vi "SetQMC_SetQMCA.vi"(0 "System no.":i32=1 min=1 step=1, 1 "Function":enum16{"SetQMC", "SetQMCA"}(ring), 2 "Axis":u8, 3 "Command":u8, 5 "error in":errorcluster, 6 "Parameter":i32, 8 "Parameter 1":u16, 9 "Parameter 2":i32) -> (14 "DLL I32 Return value":i32, 19 "error out":errorcluster)   [LabVIEW 2026]
doc: "This VI calls the SetQMC or SetQMCA function in the GCSTranslator.dll. GCSTranslator.dll and the corresponding system specific GCS DLL must be installed. The VI reads the system name from Global 2 and calls the corresponding DLL function. Parameter is only valid for SetQMC, Parameter 1 and Parameter 2 are only valid for SetQMCA. When using as a sub-VI, take special care to use the correct data representation when connecting values to the input terminals. If coercion dots appear at the terminals, the VI may not function correctly. After changing values, the update function must be called to activate the new values. See user manual for details."
uses:
  Global1.vi
  GeneralCommands/Global2 (Array).vi
panel:
  # "This vi calls the SetQMC or SetQMCA function from \nGCSTranslator.dll. GCSTranslator.dll and the corresponding \nsystem specific GCS DLL must be installed. The VI reads \nthe system name from Global 2 and calls the corresponding \nDLL function. Parameter is only valid for SetQMC, Parameter\n1 and Parameter 2 are only valid for SetQMCA."
  # "General inputs:"
  # "Function specific inputs:"
  # "Only valid for SetQMC:"
  # "Only valid for SetQMCA:"
  # "Error handling:"
  # "DLL output:"
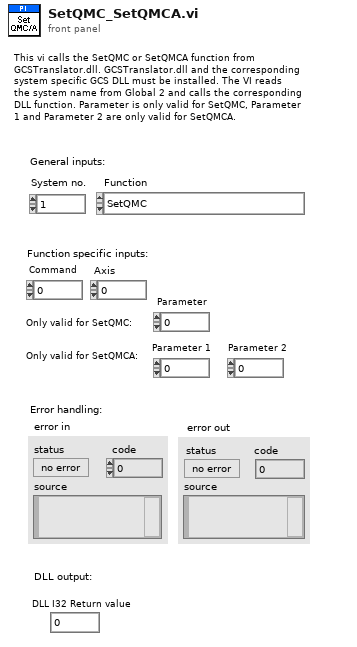
[diagram p1: front panel]
types:
  T1 = typedef "Controller names.ctl" = enum16{"None", "Analog", "C-702", "C-413", "C-414", "C-843", "C-843.PM", "C-844", "C-848", "C-865", "C-866", "C-867", "C-877", "C-880", "C-884", "C-885", "C-886", "C-887", "C-891", "E-135", "E-516", "E-517", "E-518", "E-709", "E-710", "E-712", "E-725", "E-727", "E-753", "E-754", "E-755", "E-761", "E-816", "E-861", "E-870", "E-871", "E-872", "E-873", "E-874", "F-206", "HydraPollux", "M-840", "M-850", "M-8X0", "Mercury", "Mercury_GCS", "PI_GCS2"}
  T2 = cluster{"Conn. axes":string[], "Controller name":T1}[]
  T3 = cluster{"Conn. axes":string[], "Controller name":T1}
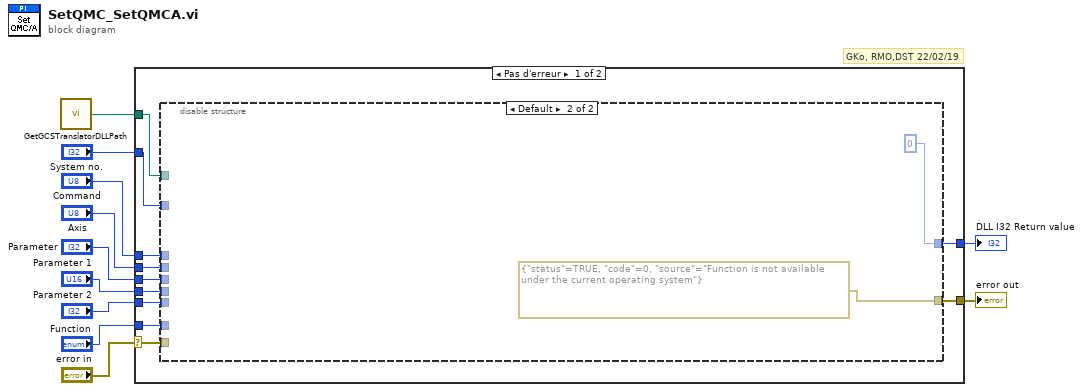
[diagram p0: block diagram]
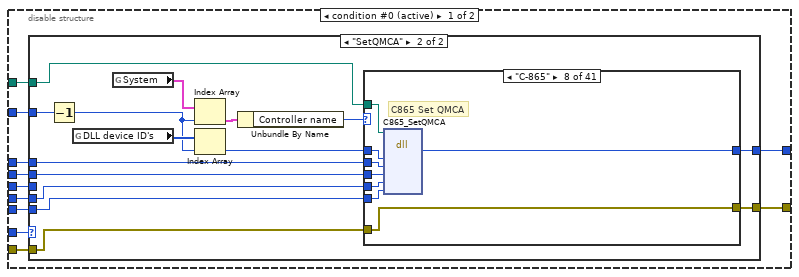
[diagram p2: hidden frame]
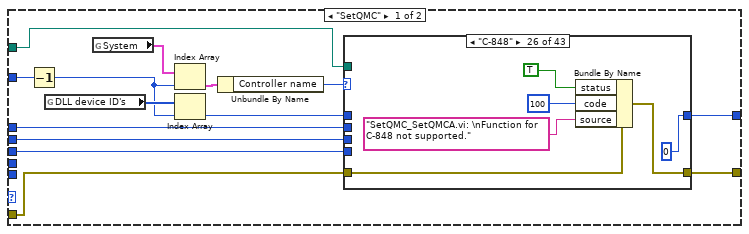
[diagram p3: hidden frame]
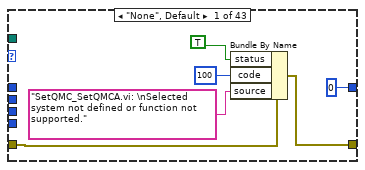
[diagram p4: hidden frame]
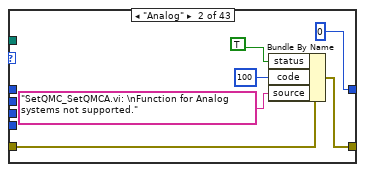
[diagram p5: hidden frame]
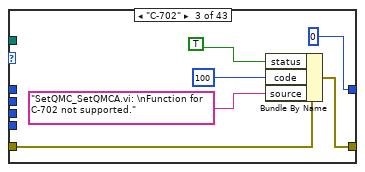
[diagram p6: hidden frame]
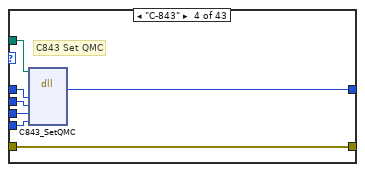
[diagram p7: hidden frame]
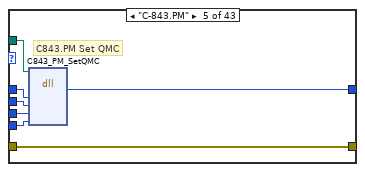
[diagram p8: hidden frame]
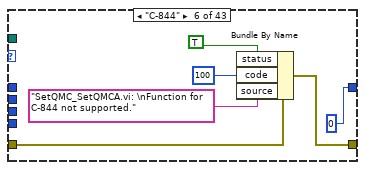
[diagram p9: hidden frame]
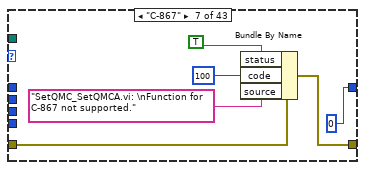
[diagram p10: hidden frame]
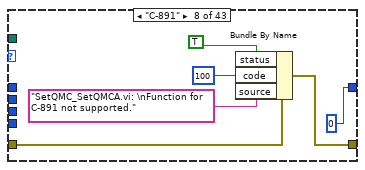
[diagram p11: hidden frame]
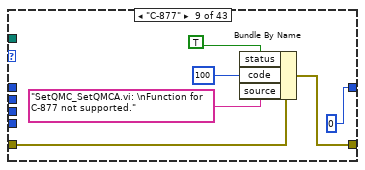
[diagram p12: hidden frame]
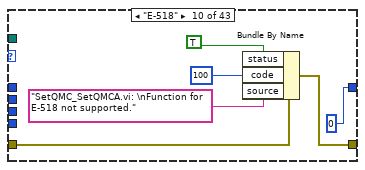
[diagram p13: hidden frame]
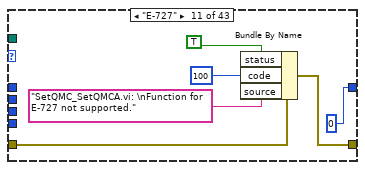
[diagram p14: hidden frame]
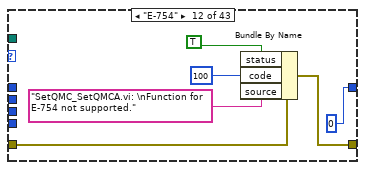
[diagram p15: hidden frame]
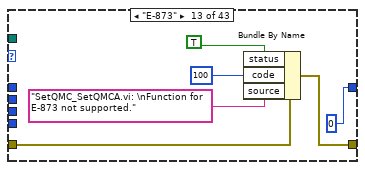
[diagram p16: hidden frame]
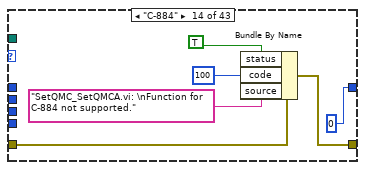
[diagram p17: hidden frame]
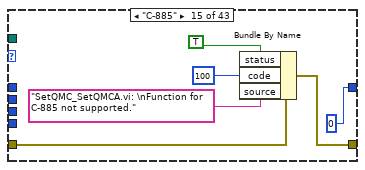
[diagram p18: hidden frame]
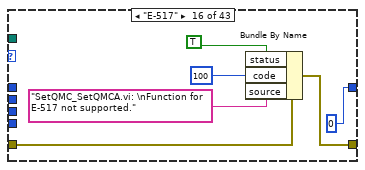
[diagram p19: hidden frame]
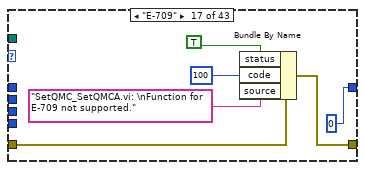
[diagram p20: hidden frame]
diagram:
  # "GKo, RMO,DST 22/02/19"
  n1 = call "GetGCSTranslatorDLLPath.vi"() -> ("DLL path"=w1:path)  [unwired: 1 in]
  n2 = case shown="Pas d'erreur" "error in" {
    selector: "error in" -> [w15 w581]
    tunnel: [w22 w581] -> w11
    tunnel: [w21 0] -> w10
    tunnel: "Command" -> [w20 _]
    tunnel: "Axis" -> [w19 _]
    tunnel: "Parameter" -> [w18 _]
    tunnel: "Parameter 1" -> [w17 _]
    tunnel: "Parameter 2" -> [w16 _]
    tunnel: "System no." -> [w14 _]
    tunnel: "Function" -> [w13 _]
    tunnel: w1 -> [w12 _]
    frame No Error {
      n3 = disable-structure shown="Default" {
        disable-tunnel: w13 -> [w33 _]
        disable-tunnel: [w32 errorcluster {"status"=TRUE, "code"=0, "source"="Function is not available under the current operating system"} ("error IO")] -> w22
        disable-tunnel: [w31 0] -> w21
        disable-tunnel: w14 -> [w30 _]
        disable-tunnel: w20 -> [w29 _]
        disable-tunnel: w19 -> [w28 _]
        disable-tunnel: w18 -> [w27 _]
        disable-tunnel: w17 -> [w26 _]
        disable-tunnel: w16 -> [w25 _]
        disable-tunnel: w15 -> [w24 _]
        disable-tunnel: w12 -> [w23 _]
        frame condition #0 (active) {
          n4 = case shown="\"SetQMCA\"" w33 {
            tunnel: w30 -> [w46 w323]
            tunnel: w24 -> [w40 w316]
            tunnel: [w39 w315] -> w32
            tunnel: [w47 w324] -> w31
            tunnel: w29 -> [w43 w320]
            tunnel: w28 -> [w42 w319]
            tunnel: w27 -> [w41 _]
            tunnel: w26 -> [_ w318]
            tunnel: w25 -> [_ w317]
            tunnel: w23 -> [w34 w310]
            frame "SetQMC" {
              n5 = Decrement(x=w46) -> (x-1=w37:i32)
              n6 = global read "Global1.vi" "DLL device ID's"() -> (w45:i32[])
              n7 = global read "Global2 (Array).vi" "System"() -> (w38:T2)
              n8 = Index Array(array=w38, index=w37) -> (element=w36:T3)
              n9 = Index Array(array=w45, index=w37) -> (element=w44:i32)
              n10 = Unbundle By Name(w36) -> ("Controller name"=w35:T1)
              n11 = case shown="\"C-848\"" w35 {
                tunnel: [0 0 0 w72 w79 0 0 0 0 0 0 0 0 0 0 0 0 0 0 0 0 0 0 0 0 0 w212 w219 0 0 0 0 0 0 0 0 0 0 0 0 0 0 0] -> w47
                tunnel: w44 -> [_ _ _ w71 w78 _ _ _ _ _ _ _ _ _ _ _ _ _ _ _ _ _ _ _ _ _ w211 w218 _ _ _ _ _ _ _ _ _ _ _ _ _ _ _]
                tunnel: w43 -> [_ _ _ w70 w77 _ _ _ _ _ _ _ _ _ _ _ _ _ _ _ _ _ _ _ _ _ w210 w217 _ _ _ _ _ _ _ _ _ _ _ _ _ _ _]
                tunnel: w42 -> [_ _ _ w69 w76 _ _ _ _ _ _ _ _ _ _ _ _ _ _ _ _ _ _ _ _ _ w209 w216 _ _ _ _ _ _ _ _ _ _ _ _ _ _ _]
                tunnel: w41 -> [_ _ _ w68 w75 _ _ _ _ _ _ _ _ _ _ _ _ _ _ _ _ _ _ _ _ _ w208 w215 _ _ _ _ _ _ _ _ _ _ _ _ _ _ _]
                tunnel: [w51 w58 w63 w67 w74 w83 w89 w95 w101 w107 w113 w119 w125 w131 w137 w143 w149 w155 w161 w167 w173 w179 w185 w191 w197 w203 w207 w214 w223 w229 w235 w241 w247 w253 w259 w265 w271 w277 w283 w289 w295 w301 w307] -> w39
                tunnel: w40 -> [w52 w54 w64 w67 w74 w84 w90 w96 w102 w108 w114 w120 w126 w132 w138 w144 w150 w156 w162 w168 w174 w180 w186 w192 w198 w204 w207 w214 w224 w230 w236 w242 w248 w254 w260 w266 w272 w278 w284 w290 w296 w302 w308]
                tunnel: w34 -> [_ _ _ w66 w73 _ _ _ _ _ _ _ _ _ _ _ _ _ _ _ _ _ _ _ _ _ w206 w213 _ _ _ _ _ _ _ _ _ _ _ _ _ _ _]
                frame "None", Default {
                  n12 = Bundle By Name(cluster=w52, "status"=TRUE, "code"=100, "source"="SetQMC_SetQMCA.vi: \nSelected system not defined or function not supported.") -> (w51:errorcluster)
                }
                frame "Analog" {
                  n13 = Bundle By Name(cluster=w54, "status"=TRUE, "code"=100, "source"="SetQMC_SetQMCA.vi: \nFunction for Analog systems not supported.") -> (w58:errorcluster)
                }
                frame "C-702" {
                  n14 = Bundle By Name(cluster=w64, "status"=TRUE, "code"=100, "source"="SetQMC_SetQMCA.vi: \nFunction for C-702 not supported.") -> (w63:errorcluster)
                }
                frame "C-843" {
                  # "C843 Set QMC"
                  n15 = dll-call lib="T:/Entwicklung/HostSoftware/LabVIEW/GCSDrivers/source/GCS2LabVIEW/Low Level/GCSTranslator.dll" fn="C843_SetQMC"(path in=w66, "ID"=w71, "Cmd"=w70, "Axis"=w69, "Param"=w68) -> ("return type"=w72:i32)  [unwired: 6 in, 2 out]
                }
                frame "C-843.PM" {
                  # "C843.PM Set QMC"
                  n16 = dll-call lib="T:/Entwicklung/HostSoftware/LabVIEW/GCSDrivers/source/GCS2LabVIEW/Low Level/GCSTranslator.dll" fn="C843_PM_SetQMC"(path in=w73, "ID"=w78, "Cmd"=w77, "Axis"=w76, "Param"=w75) -> ("return type"=w79:i32)  [unwired: 6 in, 2 out]
                }
                frame "C-844" {
                  n17 = Bundle By Name(cluster=w84, "status"=TRUE, "code"=100, "source"="SetQMC_SetQMCA.vi: \nFunction for C-844 not supported.") -> (w83:errorcluster)
                }
                frame "C-867" {
                  n18 = Bundle By Name(cluster=w90, "status"=TRUE, "code"=100, "source"="SetQMC_SetQMCA.vi: \nFunction for C-867 not supported.") -> (w89:errorcluster)
                }
                frame "C-891" {
                  n19 = Bundle By Name(cluster=w96, "status"=TRUE, "code"=100, "source"="SetQMC_SetQMCA.vi: \nFunction for C-891 not supported.") -> (w95:errorcluster)
                }
                frame "C-877" {
                  n20 = Bundle By Name(cluster=w102, "status"=TRUE, "code"=100, "source"="SetQMC_SetQMCA.vi: \nFunction for C-877 not supported.") -> (w101:errorcluster)
                }
                frame "E-518" {
                  n21 = Bundle By Name(cluster=w108, "status"=TRUE, "code"=100, "source"="SetQMC_SetQMCA.vi: \nFunction for E-518 not supported.") -> (w107:errorcluster)
                }
                frame "E-727" {
                  n22 = Bundle By Name(cluster=w114, "status"=TRUE, "code"=100, "source"="SetQMC_SetQMCA.vi: \nFunction for E-727 not supported.") -> (w113:errorcluster)
                }
                frame "E-754" {
                  n23 = Bundle By Name(cluster=w120, "status"=TRUE, "code"=100, "source"="SetQMC_SetQMCA.vi: \nFunction for E-754 not supported.") -> (w119:errorcluster)
                }
                frame "E-873" {
                  n24 = Bundle By Name(cluster=w126, "status"=TRUE, "code"=100, "source"="SetQMC_SetQMCA.vi: \nFunction for E-873 not supported.") -> (w125:errorcluster)
                }
                frame "C-884" {
                  n25 = Bundle By Name(cluster=w132, "status"=TRUE, "code"=100, "source"="SetQMC_SetQMCA.vi: \nFunction for C-884 not supported.") -> (w131:errorcluster)
                }
                frame "C-885" {
                  n26 = Bundle By Name(cluster=w138, "status"=TRUE, "code"=100, "source"="SetQMC_SetQMCA.vi: \nFunction for C-885 not supported.") -> (w137:errorcluster)
                }
                frame "E-517" {
                  n27 = Bundle By Name(cluster=w144, "status"=TRUE, "code"=100, "source"="SetQMC_SetQMCA.vi: \nFunction for E-517 not supported.") -> (w143:errorcluster)
                }
                frame "E-709" {
                  n28 = Bundle By Name(cluster=w150, "status"=TRUE, "code"=100, "source"="SetQMC_SetQMCA.vi: \nFunction for E-709 not supported.") -> (w149:errorcluster)
                }
                frame "E-712" {
                  n29 = Bundle By Name(cluster=w156, "status"=TRUE, "code"=100, "source"="SetQMC_SetQMCA.vi: \nFunction for E-712 not supported.") -> (w155:errorcluster)
                }
                frame "E-725" {
                  n30 = Bundle By Name(cluster=w162, "status"=TRUE, "code"=100, "source"="SetQMC_SetQMCA.vi: \nFunction for E-725 not supported.") -> (w161:errorcluster)
                }
                frame "E-861" {
                  n31 = Bundle By Name(cluster=w168, "status"=TRUE, "code"=100, "source"="SetQMC_SetQMCA.vi: \nFunction for E-861 not supported.") -> (w167:errorcluster)
                }
                frame "E-870" {
                  n32 = Bundle By Name(cluster=w174, "status"=TRUE, "code"=100, "source"="SetQMC_SetQMCA.vi: \nFunction for E-870 not supported.") -> (w173:errorcluster)
                }
                frame "E-871" {
                  n33 = Bundle By Name(cluster=w180, "status"=TRUE, "code"=100, "source"="SetQMC_SetQMCA.vi: \nFunction for E-871 not supported.") -> (w179:errorcluster)
                }
                frame "HydraPollux" {
                  n34 = Bundle By Name(cluster=w186, "status"=TRUE, "code"=100, "source"="SetQMC_SetQMCA.vi: \nFunction for Hydra/Pollux not supported.") -> (w185:errorcluster)
                }
                frame "Mercury_GCS" {
                  n35 = Bundle By Name(cluster=w192, "status"=TRUE, "code"=100, "source"="SetQMC_SetQMCA.vi: \nFunction for Mercury_GCS not supported.") -> (w191:errorcluster)
                }
                frame "C-413" {
                  n36 = Bundle By Name(cluster=w198, "status"=TRUE, "code"=100, "source"="SetQMC_SetQMCA.vi: \nFunction for C-413 not supported.") -> (w197:errorcluster)
                }
                frame "C-848" {
                  n37 = Bundle By Name(cluster=w204, "status"=TRUE, "code"=100, "source"="SetQMC_SetQMCA.vi: \nFunction for C-848 not supported.") -> (w203:errorcluster)
                }
                frame "C-865" {
                  # "C865 Set QMC"
                  n38 = dll-call lib="T:/Entwicklung/HostSoftware/LabVIEW/GCSDrivers/source/GCS2LabVIEW/Low Level/GCSTranslator.dll" fn="C865_SetQMC"(path in=w206, "ID"=w211, "Cmd"=w210, "Axis"=w209, "Param"=w208) -> ("return type"=w212:i32)  [unwired: 6 in, 2 out]
                }
                frame "C-866" {
                  # "C866 Set QMC"
                  n39 = dll-call lib="T:/Entwicklung/HostSoftware/LabVIEW/GCSDrivers/source/GCS2LabVIEW/Low Level/GCSTranslator.dll" fn="SetQMC"(path in=w213, "ID"=w218, "Cmd"=w217, "Axis"=w216, "Param"=w215) -> ("return type"=w219:i32)  [unwired: 6 in, 2 out]
                }
                frame "C-880" {
                  n40 = Bundle By Name(cluster=w224, "status"=TRUE, "code"=100, "source"="SetQMC_SetQMCA.vi: \nFunction for C-880 not supported.") -> (w223:errorcluster)
                }
                frame "E-516" {
                  n41 = Bundle By Name(cluster=w230, "status"=TRUE, "code"=100, "source"="SetQMC_SetQMCA.vi: \nFunction for E-516 not supported.") -> (w229:errorcluster)
                }
                frame "E-710" {
                  n42 = Bundle By Name(cluster=w236, "status"=TRUE, "code"=100, "source"="SetQMC_SetQMCA.vi: \nFunction for E-710 not supported.") -> (w235:errorcluster)
                }
                frame "E-872" {
                  n43 = Bundle By Name(cluster=w242, "status"=TRUE, "code"=100, "source"="SetQMC_SetQMCA.vi: \nFunction for E-872 not supported.") -> (w241:errorcluster)
                }
                frame "E-874" {
                  n44 = Bundle By Name(cluster=w248, "status"=TRUE, "code"=100, "source"="SetQMC_SetQMCA.vi: \nFunction for E-874 not supported.") -> (w247:errorcluster)
                }
                frame "PI_GCS2" {
                  n45 = Bundle By Name(cluster=w254, "status"=TRUE, "code"=100, "source"="SetQMC_SetQMCA.vi: \nFunction for PI_GCS_2 not supported.") -> (w253:errorcluster)
                }
                frame "E-753" {
                  n46 = Bundle By Name(cluster=w260, "status"=TRUE, "code"=100, "source"="SetQMC_SetQMCA.vi: \nFunction for E-753 not supported.") -> (w259:errorcluster)
                }
                frame "E-755" {
                  n47 = Bundle By Name(cluster=w266, "status"=TRUE, "code"=100, "source"="SetQMC_SetQMCA.vi: \nFunction for E-755 not supported.") -> (w265:errorcluster)
                }
                frame "E-761" {
                  n48 = Bundle By Name(cluster=w272, "status"=TRUE, "code"=100, "source"="SetQMC_SetQMCA.vi: \nFunction for E-761 not supported.") -> (w271:errorcluster)
                }
                frame "E-816" {
                  n49 = Bundle By Name(cluster=w278, "status"=TRUE, "code"=100, "source"="SetQMC_SetQMCA.vi: \nFunction for E-816 not supported.") -> (w277:errorcluster)
                }
                frame "F-206" {
                  n50 = Bundle By Name(cluster=w284, "status"=TRUE, "code"=100, "source"="SetQMC_SetQMCA.vi: \nFunction for F-206 not supported.") -> (w283:errorcluster)
                }
                frame "M-840" {
                  n51 = Bundle By Name(cluster=w290, "status"=TRUE, "code"=100, "source"="SetQMC_SetQMCA.vi: \nFunction for M-840 not supported.") -> (w289:errorcluster)
                }
                frame "M-850" {
                  n52 = Bundle By Name(cluster=w296, "status"=TRUE, "code"=100, "source"="SetQMC_SetQMCA.vi: \nFunction for M-850 not supported.") -> (w295:errorcluster)
                }
                frame "M-8X0" {
                  n53 = Bundle By Name(cluster=w302, "status"=TRUE, "code"=100, "source"="SetQMC_SetQMCA.vi: \nFunction for M-8X0 not supported.") -> (w301:errorcluster)
                }
                frame "Mercury" {
                  n54 = Bundle By Name(cluster=w308, "status"=TRUE, "code"=100, "source"="SetQMC_SetQMCA.vi: \nFunction for Mercury not supported.") -> (w307:errorcluster)
                }
              }
            }
            frame "SetQMCA" {
              n55 = Decrement(x=w323) -> (x-1=w313:i32)
              n56 = global read "Global1.vi" "DLL device ID's"() -> (w322:i32[])
              n57 = global read "Global2 (Array).vi" "System"() -> (w314:T2)
              n58 = Index Array(array=w314, index=w313) -> (element=w312:T3)
              n59 = Index Array(array=w322, index=w313) -> (element=w321:i32)
              n60 = Unbundle By Name(w312) -> ("Controller name"=w311:T1)
              n61 = case shown="\"C-865\"" w311 {
                tunnel: [0 0 0 w350 w358 0 0 w378 w386 0 0 0 0 0 0 0 0 0 0 0 0 0 0 0 0 0 0 0 0 0 0 0 0 0 0 0 0 0 0 0 0] -> w324
                tunnel: w321 -> [_ _ _ w349 w357 _ _ w377 w385 _ _ _ _ _ _ _ _ _ _ _ _ _ _ _ _ _ _ _ _ _ _ _ _ _ _ _ _ _ _ _ _]
                tunnel: w320 -> [_ _ _ w348 w356 _ _ w376 w384 _ _ _ _ _ _ _ _ _ _ _ _ _ _ _ _ _ _ _ _ _ _ _ _ _ _ _ _ _ _ _ _]
                tunnel: w319 -> [_ _ _ w347 w355 _ _ w375 w383 _ _ _ _ _ _ _ _ _ _ _ _ _ _ _ _ _ _ _ _ _ _ _ _ _ _ _ _ _ _ _ _]
                tunnel: w317 -> [_ _ _ w346 w354 _ _ w374 w382 _ _ _ _ _ _ _ _ _ _ _ _ _ _ _ _ _ _ _ _ _ _ _ _ _ _ _ _ _ _ _ _]
                tunnel: w318 -> [_ _ _ w345 w353 _ _ w373 w381 _ _ _ _ _ _ _ _ _ _ _ _ _ _ _ _ _ _ _ _ _ _ _ _ _ _ _ _ _ _ _ _]
                tunnel: w316 -> [w326 w332 w338 w344 w352 w360 w366 w372 w380 w388 w394 w400 w406 w412 w418 w424 w430 w436 w442 w448 w454 w460 w466 w472 w478 w484 w490 w496 w502 w508 w514 w520 w526 w532 w538 w544 w550 w556 w562 w568 w574]
                tunnel: [w325 w331 w337 w344 w352 w359 w365 w372 w380 w387 w393 w399 w405 w411 w417 w423 w429 w435 w441 w447 w453 w459 w465 w471 w477 w483 w489 w495 w501 w507 w513 w519 w525 w531 w537 w543 w549 w555 w561 w567 w573] -> w315
                tunnel: w310 -> [_ _ _ w343 w351 _ _ w371 w379 _ _ _ _ _ _ _ _ _ _ _ _ _ _ _ _ _ _ _ _ _ _ _ _ _ _ _ _ _ _ _ _]
                frame "None", Default {
                  n62 = Bundle By Name(cluster=w326, "status"=TRUE, "code"=100, "source"="SetQMC_SetQMCA.vi: \nSelected system not defined or function not supported.") -> (w325:errorcluster)
                }
                frame "Analog" {
                  n63 = Bundle By Name(cluster=w332, "status"=TRUE, "code"=100, "source"="SetQMC_SetQMCA.vi: \nFunction for Analog systems not supported.") -> (w331:errorcluster)
                }
                frame "C-702" {
                  n64 = Bundle By Name(cluster=w338, "status"=TRUE, "code"=100, "source"="SetQMC_SetQMCA.vi: \nFunction for C-702 not supported.") -> (w337:errorcluster)
                }
                frame "C-843" {
                  # "C843 Set QMCA"
                  n65 = dll-call lib="T:/Entwicklung/HostSoftware/LabVIEW/GCSDrivers/source/GCS2LabVIEW/Low Level/GCSTranslator.dll" fn="C843_SetQMCA"(path in=w343, "ID"=w349, "Cmd"=w348, "Axis"=w347, "Param1"=w345, "lParam2"=w346) -> ("return type"=w350:i32)  [unwired: 7 in, 2 out]
                }
                frame "C-843.PM" {
                  # "C843.PM Set QMCA"
                  n66 = dll-call lib="T:/Entwicklung/HostSoftware/LabVIEW/GCSDrivers/source/GCS2LabVIEW/Low Level/GCSTranslator.dll" fn="C843_PM_SetQMCA"(path in=w351, "ID"=w357, "Cmd"=w356, "Axis"=w355, "Param1"=w353, "lParam2"=w354) -> ("return type"=w358:i32)  [unwired: 7 in, 2 out]
                }
                frame "C-844" {
                  n67 = Bundle By Name(cluster=w360, "status"=TRUE, "code"=100, "source"="SetQMC_SetQMCA.vi: \nFunction for C-844 not supported.") -> (w359:errorcluster)
                }
                frame "C-848" {
                  n68 = Bundle By Name(cluster=w366, "status"=TRUE, "code"=100, "source"="SetQMC_SetQMCA.vi: \nFunction for C-848 not supported.") -> (w365:errorcluster)
                }
                frame "C-865" {
                  # "C865 Set QMCA"
                  n69 = dll-call lib="T:/Entwicklung/HostSoftware/LabVIEW/GCSDrivers/source/GCS2LabVIEW/Low Level/GCSTranslator.dll" fn="C865_SetQMCA"(path in=w371, "ID"=w377, "Cmd"=w376, "Axis"=w375, "Param1"=w373, "lParam2"=w374) -> ("return type"=w378:i32)  [unwired: 7 in, 2 out]
                }
                frame "C-866" {
                  # "C866 Set QMCA"
                  n70 = dll-call lib="T:/Entwicklung/HostSoftware/LabVIEW/GCSDrivers/source/GCS2LabVIEW/Low Level/GCSTranslator.dll" fn="SetQMCA"(path in=w379, "ID"=w385, "Cmd"=w384, "Axis"=w383, "Param1"=w381, "lParam2"=w382) -> ("return type"=w386:i32)  [unwired: 7 in, 2 out]
                }
                frame "C-880" {
                  n71 = Bundle By Name(cluster=w388, "status"=TRUE, "code"=100, "source"="SetQMC_SetQMCA.vi: \nFunction for C-880 not supported.") -> (w387:errorcluster)
                }
                frame "E-516" {
                  n72 = Bundle By Name(cluster=w394, "status"=TRUE, "code"=100, "source"="SetQMC_SetQMCA.vi: \nFunction for E-516 not supported.") -> (w393:errorcluster)
                }
                frame "E-710" {
                  n73 = Bundle By Name(cluster=w400, "status"=TRUE, "code"=100, "source"="SetQMC_SetQMCA.vi: \nFunction for E-710 not supported.") -> (w399:errorcluster)
                }
                frame "E-753" {
                  n74 = Bundle By Name(cluster=w406, "status"=TRUE, "code"=100, "source"="SetQMC_SetQMCA.vi: \nFunction for E-753 not supported.") -> (w405:errorcluster)
                }
                frame "E-755" {
                  n75 = Bundle By Name(cluster=w412, "status"=TRUE, "code"=100, "source"="SetQMC_SetQMCA.vi: \nFunction for E-755 not supported.") -> (w411:errorcluster)
                }
                frame "E-761" {
                  n76 = Bundle By Name(cluster=w418, "status"=TRUE, "code"=100, "source"="SetQMC_SetQMCA.vi: \nFunction for E-761 not supported.") -> (w417:errorcluster)
                }
                frame "E-816" {
                  n77 = Bundle By Name(cluster=w424, "status"=TRUE, "code"=100, "source"="SetQMC_SetQMCA.vi: \nFunction for E-816 not supported.") -> (w423:errorcluster)
                }
                frame "F-206" {
                  n78 = Bundle By Name(cluster=w430, "status"=TRUE, "code"=100, "source"="SetQMC_SetQMCA.vi: \nFunction for F-206 not supported.") -> (w429:errorcluster)
                }
                frame "HydraPollux" {
                  n79 = Bundle By Name(cluster=w436, "status"=TRUE, "code"=100, "source"="SetQMC_SetQMCA.vi: \nFunction for Hydra/Pollux  not supported.") -> (w435:errorcluster)
                }
                frame "Mercury_GCS" {
                  n80 = Bundle By Name(cluster=w442, "status"=TRUE, "code"=100, "source"="SetQMC_SetQMCA.vi: \nFunction for Mercury_GCS  not supported.") -> (w441:errorcluster)
                }
                frame "C-413" {
                  n81 = Bundle By Name(cluster=w448, "status"=TRUE, "code"=100, "source"="SetQMC_SetQMCA.vi: \nFunction for C-413  not supported.") -> (w447:errorcluster)
                }
                frame "C-867" {
                  n82 = Bundle By Name(cluster=w454, "status"=TRUE, "code"=100, "source"="SetQMC_SetQMCA.vi: \nFunction for C-867  not supported.") -> (w453:errorcluster)
                }
                frame "C-891" {
                  n83 = Bundle By Name(cluster=w460, "status"=TRUE, "code"=100, "source"="SetQMC_SetQMCA.vi: \nFunction for C-891  not supported.") -> (w459:errorcluster)
                }
                frame "C-885" {
                  n84 = Bundle By Name(cluster=w466, "status"=TRUE, "code"=100, "source"="SetQMC_SetQMCA.vi: \nFunction for C-885  not supported.") -> (w465:errorcluster)
                }
                frame "C-884" {
                  n85 = Bundle By Name(cluster=w472, "status"=TRUE, "code"=100, "source"="SetQMC_SetQMCA.vi: \nFunction for C-884  not supported.") -> (w471:errorcluster)
                }
                frame "E-517" {
                  n86 = Bundle By Name(cluster=w478, "status"=TRUE, "code"=100, "source"="SetQMC_SetQMCA.vi: \nFunction for E-517  not supported.") -> (w477:errorcluster)
                }
                frame "E-709" {
                  n87 = Bundle By Name(cluster=w484, "status"=TRUE, "code"=100, "source"="SetQMC_SetQMCA.vi: \nFunction for E-709  not supported.") -> (w483:errorcluster)
                }
                frame "E-712" {
                  n88 = Bundle By Name(cluster=w490, "status"=TRUE, "code"=100, "source"="SetQMC_SetQMCA.vi: \nFunction for E-712  not supported.") -> (w489:errorcluster)
                }
                frame "E-725" {
                  n89 = Bundle By Name(cluster=w496, "status"=TRUE, "code"=100, "source"="SetQMC_SetQMCA.vi: \nFunction for E-725  not supported.") -> (w495:errorcluster)
                }
                frame "E-861" {
                  n90 = Bundle By Name(cluster=w502, "status"=TRUE, "code"=100, "source"="SetQMC_SetQMCA.vi: \nFunction for E-861  not supported.") -> (w501:errorcluster)
                }
                frame "E-870" {
                  n91 = Bundle By Name(cluster=w508, "status"=TRUE, "code"=100, "source"="SetQMC_SetQMCA.vi: \nFunction for E-870  not supported.") -> (w507:errorcluster)
                }
                frame "E-871" {
                  n92 = Bundle By Name(cluster=w514, "status"=TRUE, "code"=100, "source"="SetQMC_SetQMCA.vi: \nFunction for E-871  not supported.") -> (w513:errorcluster)
                }
                frame "E-873" {
                  n93 = Bundle By Name(cluster=w520, "status"=TRUE, "code"=100, "source"="SetQMC_SetQMCA.vi: \nFunction for E-873  not supported.") -> (w519:errorcluster)
                }
                frame "PI_GCS2" {
                  n94 = Bundle By Name(cluster=w526, "status"=TRUE, "code"=100, "source"="SetQMC_SetQMCA.vi: \nFunction for PI_GCS_2  not supported.") -> (w525:errorcluster)
                }
                frame "C-877" {
                  n95 = Bundle By Name(cluster=w532, "status"=TRUE, "code"=100, "source"="SetQMC_SetQMCA.vi: \nFunction for C-877  not supported.") -> (w531:errorcluster)
                }
                frame "E-518" {
                  n96 = Bundle By Name(cluster=w538, "status"=TRUE, "code"=100, "source"="SetQMC_SetQMCA.vi: \nFunction for E-518  not supported.") -> (w537:errorcluster)
                }
                frame "E-727" {
                  n97 = Bundle By Name(cluster=w544, "status"=TRUE, "code"=100, "source"="SetQMC_SetQMCA.vi: \nFunction for E-727  not supported.") -> (w543:errorcluster)
                }
                frame "E-754" {
                  n98 = Bundle By Name(cluster=w550, "status"=TRUE, "code"=100, "source"="SetQMC_SetQMCA.vi: \nFunction for E-754  not supported.") -> (w549:errorcluster)
                }
                frame "M-840" {
                  n99 = Bundle By Name(cluster=w556, "status"=TRUE, "code"=100, "source"="SetQMC_SetQMCA.vi: \nFunction for M-840 not supported.") -> (w555:errorcluster)
                }
                frame "M-850" {
                  n100 = Bundle By Name(cluster=w562, "status"=TRUE, "code"=100, "source"="SetQMC_SetQMCA.vi: \nFunction for M-850 not supported.") -> (w561:errorcluster)
                }
                frame "M-8X0" {
                  n101 = Bundle By Name(cluster=w568, "status"=TRUE, "code"=100, "source"="SetQMC_SetQMCA.vi: \nFunction for M-8X0 not supported.") -> (w567:errorcluster)
                }
                frame "Mercury" {
                  n102 = Bundle By Name(cluster=w574, "status"=TRUE, "code"=100, "source"="SetQMC_SetQMCA.vi: \nFunction for Mercury not supported.") -> (w573:errorcluster)
                }
              }
            }
          }
        }
        frame condition #1 {
        }
      }
    }
    frame Error {
    }
  }
  "error out" <- w11
  "DLL I32 Return value" <- w10
